vi "XML Script - GenericSubVI (Refnum).vi"(0 "name":string, 1 "prefix (name)":string, 2 "path (VI Refnum)":refnum<vi>, 3 "instantiation path (VI Refnum)":refnum<vi>, 5 "in":i32=-1) -> (6 "XML Script Command - SubVI":string, 9 "name (wire source)":string)   [LabVIEW 2017]
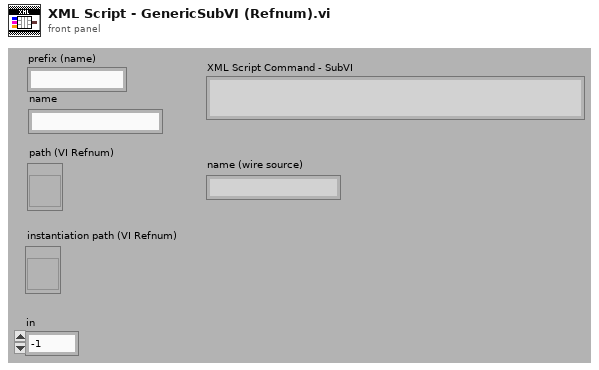
[diagram p1: front panel]
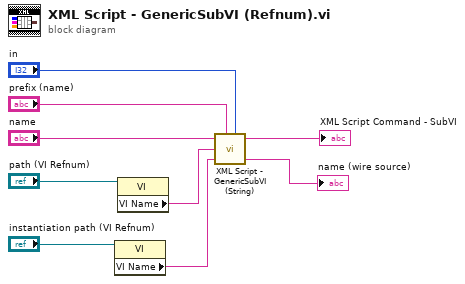
[diagram p0: block diagram]
diagram:
  n1 = property class="VI"(reference="instantiation path (VI Refnum)") -> ("VI Name"=w1:string)  [unwired: 1 in, 2 out]
  n2 = property class="VI"(reference="path (VI Refnum)") -> ("VI Name"=w3:string)  [unwired: 1 in, 2 out]
  n3 = call <vilib>:"XML Script - GenericSubVI (String).vi"("name"="name", "prefix (name)"="prefix (name)", "path"=w3, "instantiationPath"=w1, "in"="in") -> ("XML Script Command - SubVI"=→"XML Script Command - SubVI":string, "name (wire source)"=→"name (wire source)":string)  [unwired: 1 in, 2 out]
